vi "Implicit Timing Wrapper.vi"(0 "Task map in":map{string, refnum<k21>}(c390), 5 "Message Data in":T2, 11 "error in (no error)":errorcluster) -> (4 "Task map out":map{string, refnum<k21>}(c390), 6 "Message Data out":T1, 15 "error out":errorcluster)   [LabVIEW 2021, in "NI DAQmx_wrapper.lvlib"]
uses:
  NI DAQmx_wrapper.lvlib
  NI DAQmx_server/RPC Messages/nidaqmx_grpc_CfgImplicitTimingRequest.ctl
  NI DAQmx_server/RPC Messages/nidevice_grpc_Session_session/nidevice_grpc_Session_session.lvclass
  NI DAQmx_server/RPC Messages/nidaqmx_grpc_CfgImplicitTimingRequest_sample_mode_enum/nidaqmx_grpc_CfgImplicitTimingRequest_sample_mode_enum.lvclass
  NI DAQmx_server/RPC Messages/nidevice_grpc_Session.ctl
  NI DAQmx_server/RPC Messages/nidaqmx_grpc_CfgImplicitTimingResponse.ctl
  NI DAQmx_server/RPC Messages/nidaqmx_grpc_CfgImplicitTimingRequest_sample_mode_enum/nidaqmx_grpc_CfgImplicitTimingRequest_sample_mode_enum.lvclass/nidaqmx_grpc_CfgImplicitTimingRequest_sample_mode_enum.ctl
  NI DAQmx_server/RPC Messages/nidevice_grpc_Session_session/nidevice_grpc_Session_session.lvclass/nidevice_grpc_Session_session.ctl
  <vilib>/DAQmx/configure/timing.llb/DAQmx Timing (Implicit).vi
  NI DAQmx_server/NI DAQmx_server.lvlib
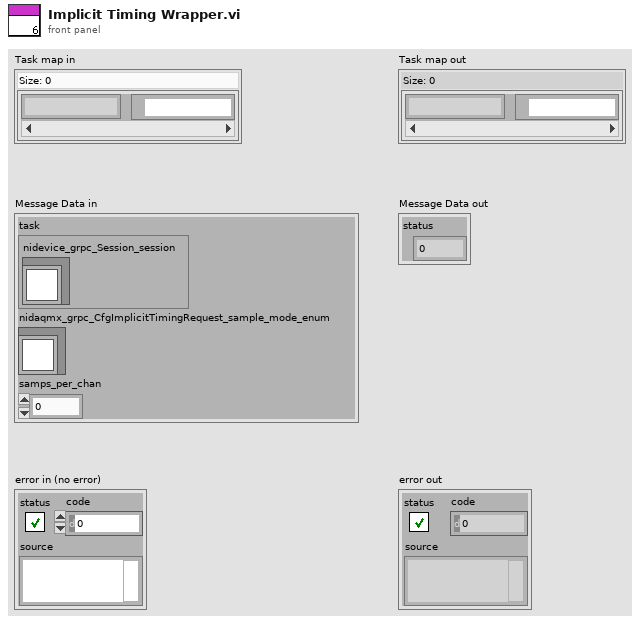
[diagram p1: front panel]
types:
  T1 = typedef "NI DAQmx_server.lvlib/nidaqmx_grpc_CfgImplicitTimingResponse.ctl" = cluster{"status":i32}
  T2 = typedef "NI DAQmx_server.lvlib/nidaqmx_grpc_CfgImplicitTimingRequest.ctl" = cluster{"task":T3, "nidaqmx_grpc_CfgImplicitTimingRequest_sample_mode_enum":refnum<class "nidaqmx_grpc_CfgImplicitTimingRequest_sample_mode_enum.lvclass">, "samps_per_chan":u64}
  T3 = typedef "NI DAQmx_server.lvlib/nidevice_grpc_Session.ctl" = cluster{"nidevice_grpc_Session_session":refnum<class "nidevice_grpc_Session_session.lvclass">}
  T4 = typedef "NI DAQmx_server.lvlib/nidaqmx_grpc_AcquisitionType.ctl" = enum32{"ACQUISITION_TYPE_UNSPECIFIED", "ACQUISITION_TYPE_FINITE_SAMPS", "ACQUISITION_TYPE_CONT_SAMPS", "ACQUISITION_TYPE_HW_TIMED_SINGLE_POINT"}
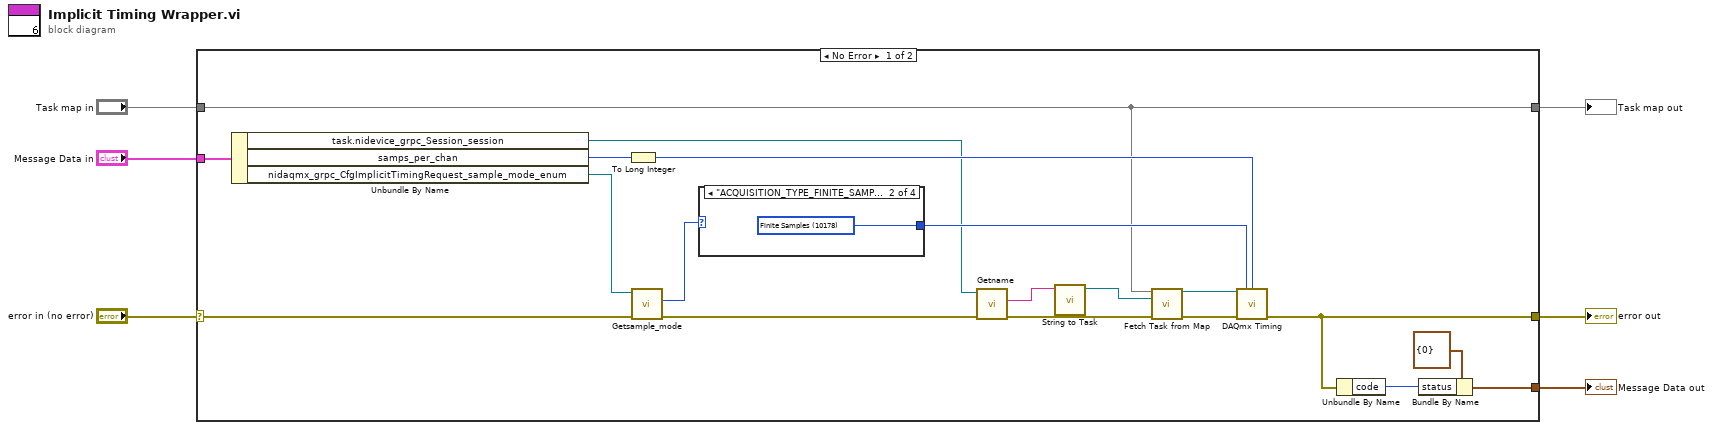
[diagram p0: block diagram]
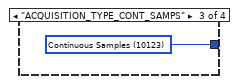
[diagram p3: hidden frame]
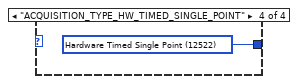
[diagram p4: hidden frame]
diagram:
  n1 = case shown="No Error" "error in (no error)" {
    selector: "error in (no error)" -> [w24 w30]
    tunnel: [w9 w30] -> w5
    tunnel: "Task map in" -> [w11 w29]
    tunnel: [w11 w29] -> w3
    tunnel: "Message Data in" -> [w25 _]
    tunnel: [w7 _] -> w1
    frame No Error {
      n2 = Unbundle By Name(w25) -> ("task.nidevice_grpc_Session_session"=w12:refnum<class "nidevice_grpc_Session_session.lvclass">, "samps_per_chan"=w20:u64, "nidaqmx_grpc_CfgImplicitTimingRequest_sample_mode_enum"=w23:refnum<class "nidaqmx_grpc_CfgImplicitTimingRequest_sample_mode_enum.lvclass">)
      n3 = To Long Integer(number=w20) -> (32bit integer=w19:i32)
      n4 = call "Getsample_mode.vi"("error in (no error)"=w24, "OneOfTemplate in"=w23) -> ("error out"=w16:errorcluster, "Get_Val"=w22:T4)  [unwired: 7 in, 1 out]
      n5 = case shown="\"ACQUISITION_TYPE_FINITE_SAMPS\"" w22 {
        tunnel: [_ w26 w27 w28] -> w21
        frame "ACQUISITION_TYPE_UNSPECIFIED", Default {
        }
        frame "ACQUISITION_TYPE_FINITE_SAMPS" {
          w26 = 10178 items=["Finite Samples"=10178, "Continuous Samples"=10123, "Hardware Timed Single Point"=12522] ("sample mode")
        }
        frame "ACQUISITION_TYPE_CONT_SAMPS" {
          w27 = 10123 items=["Finite Samples"=10178, "Continuous Samples"=10123, "Hardware Timed Single Point"=12522] ("sample mode")
        }
        frame "ACQUISITION_TYPE_HW_TIMED_SINGLE_POINT" {
          w28 = 12522 items=["Finite Samples"=10178, "Continuous Samples"=10123, "Hardware Timed Single Point"=12522] ("sample mode")
        }
      }
      n6 = call "Getname.vi"("error in (no error)"=w16, "OneOfTemplate in"=w12) -> ("error out"=w15:errorcluster, "Get_Val"=w18:string)  [unwired: 7 in, 1 out]
      n7 = call "String to Task.vi"("Get_Val"=w18) -> ("Refnum out"=w17:refnum<k21>)  [unwired: 10 in]
      n8 = call "Fetch Task from Map.vi"("Task map in"=w11, "Task in"=w17, "error in (no error)"=w15) -> ("Task out"=w13:refnum<k21>, "error out"=w14:errorcluster)  [unwired: 11 in]
      n9 = call-poly <vilib>:"DAQmx Timing.vi"("task/channels in"=w13, "sample mode"=w21, "samples per channel"=w19, "error in"=w14) -> ("error out"=w9:errorcluster)  [unwired: 10 in, 1 out]
      n10 = Unbundle By Name(w9) -> ("code"=w10:i32)
      n11 = Bundle By Name(cluster=T1 {"status"=0} ("Message Data"), "status"=w10) -> (w7:T1)
    }
    frame Error {
    }
  }
  "error out" <- w5
  "Task map out" <- w3
  "Message Data out" <- w1
